vi "Actor Core.vi"(8 "error in":errorcluster, 11 "Panel in":refnum<class "Sample Panel.lvclass">) -> (0 "error out":errorcluster, 3 "Actor out":refnum<class "Actor.lvclass">)   [LabVIEW 2020, in "2. Basic Panel Actors.lvlib" / "Sample Panel.lvclass"]
doc: "Shows the Label and a log of all events for the panel.\n----\nCopyright: MGI 2016\nAuthor: Derek Trepanier"
uses:
  Sample Panel.lvclass
  C:/Program Files/National Instruments/LabVIEW 2020/vi.lib/MGI/Monitored Actor/Monitored Actor/Monitored Actor/Monitored Actor.lvclass
  C:/Program Files/National Instruments/LabVIEW 2020/vi.lib/MGI/Panel Manager/Panel Actor/Panel Actor/Panel Actor.lvclass
  <vilib>/ActorFramework/Actor/Actor.lvclass
  <vilib>/ActorFramework/Message Enqueuer/Message Enqueuer.lvclass/Message Enqueuer.ctl
  <vilib>/ActorFramework/Message Enqueuer/Enqueue.vi
  <vilib>/ActorFramework/Stop Msg/Stop Msg.lvclass
  C:/Program Files/National Instruments/LabVIEW 2020/vi.lib/ActorFramework/Message/Message.lvclass
  <vilib>/ActorFramework/Message Priority Queue/Priority Enqueue.vi
  <vilib>/MGI/Panel Manager/Panel Actor/Panel Actor/Panel Actor.lvclass
  <vilib>/MGI/Monitored Actor/Monitored Actor/Monitored Actor/Monitored Actor.lvclass
panel:
  out "Label":string
  out "Top Level Panel":string
  in  "Show":bool
  in  "My Event Log":i32(listbox)
  in  "Show Dialog":bool
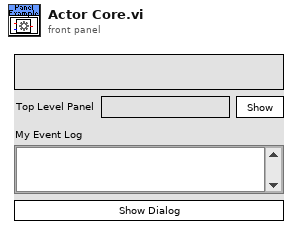
[diagram p1: front panel]
types:
  T1 = typedef "Panel.lvlib/Panel Helper.lvclass/Events.ctl" = enum16{"Initialized", "Shown", "Hidden", "Closed"}
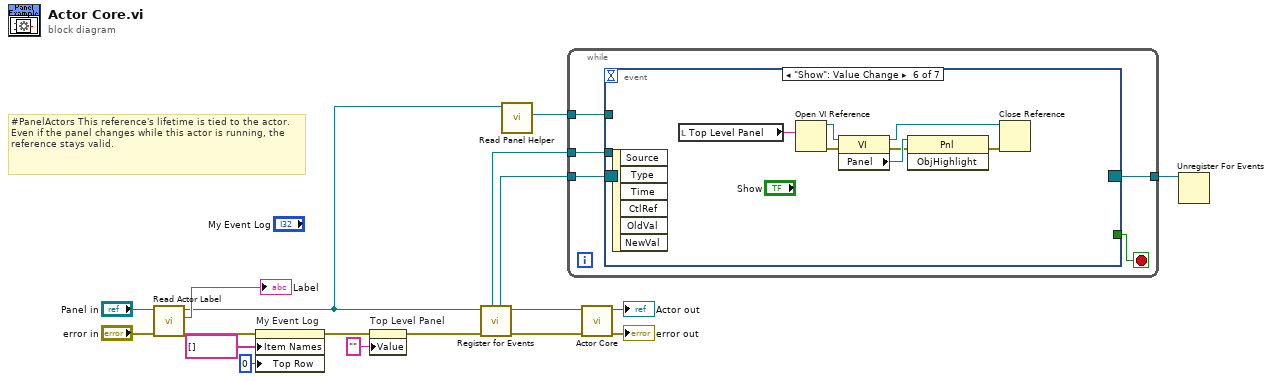
[diagram p0: block diagram]
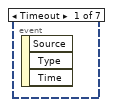
[diagram p2: hidden frame]
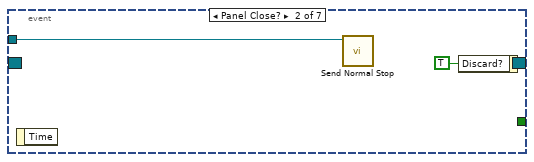
[diagram p3: hidden frame]
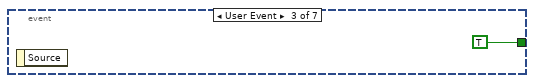
[diagram p4: hidden frame]
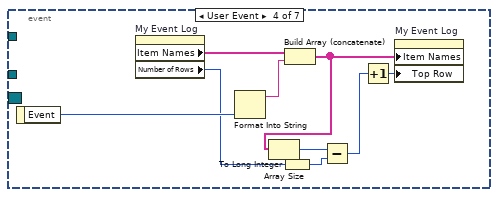
[diagram p5: hidden frame]
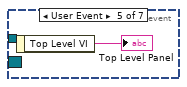
[diagram p6: hidden frame]
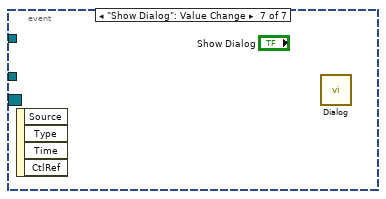
[diagram p7: hidden frame]
diagram:
  # "#PanelActors This reference's lifetime is tied to the actor. Even if the panel changes while this actor is running, the reference stays valid."
  n1 = call <vilib>:"Read Actor Label.vi"("error in (no error)"="error in", "Monitored Actor in"="Panel in") -> ("error out"=w11:errorcluster, "Actor Label"=→"Label":string, "Monitored Actor out"=w8:refnum<class "Sample Panel.lvclass">)  [unwired: 7 in]
  n2 = property on="My Event Log" class="LstBox (strict)"(error in=w11, "Item Names"=string[] [], "Top Row"=0) -> (error out=w3:errorcluster)  [unwired: 1 in, 1 out]
  n3 = property on="Top Level Panel" class="Str"(error in=w3, "Value"="" ("Top Level Panel")) -> (error out=w2:errorcluster)  [unwired: 1 in, 1 out]
  n4 = call <vilib>:"Register for Events.vi"("Error In"=w2, "Panel Actor in"=w8) -> ("Error Out"=w9:errorcluster, "Panel Actor out"=w13:refnum<class "Sample Panel.lvclass">, "Pnl Actor"=w10:refnum<event-registration>, "Self Enqueuer"=w12:refnum<class "Message Enqueuer.lvclass">)  [unwired: 6 in]
  n5 = call <vilib>:"Read Panel Helper.vi"("Panel Actor in"=w8) -> ("Panel Helper"=w7:refnum<class "Panel Helper.lvclass">)  [unwired: 9 in, 1 out]
  n6 = while {
    tunnel: w12 -> [w23]
    tunnel: w10 -> [w22]
    tunnel: w7 -> [w20]
    tunnel: [w19] -> w6
    stop <- w21 stop-if-true
    n7 = event shown="[5] \"Show\": Value Change" {
      selector: w22 -> [_ _ _ _ _ _ _]
      dyn-events: [_ _ _ _ _ _ _] -> w19
      timeout: _ -> [_ _ _ _ _ _ _]
      tunnel: w23 -> [_ w24 _ _ _ _ _]
      tunnel: [_ _ TRUE _ _ _ _] -> w21
      tunnel: w20 -> [_ _ _ _ _ _ _]
      event Timeout {
        n8 = event-data() -> ()  [unwired: 1 in, 3 out]
      }
      event Panel Close? {
        n9 = event-data() -> ()  [unwired: 1 in, 1 out]
        n10 = call <vilib>:"Send Normal Stop.vi"("Message Enqueuer"=w24) -> ()  [unwired: 10 in, 1 out]
        n11 = event-data("Discard?"=TRUE) -> ()  [unwired: 1 in, 1 out]
      }
      event User Event {
        n12 = event-data() -> ()  [unwired: 1 in, 1 out]
      }
      event User Event {
        n13 = event-data() -> ("Event"=w34:T1)  [unwired: 1 in]
        n14 = property on="My Event Log" class="LstBox (strict)"() -> ("Item Names"=w33:string[], "Number of Rows"=w31:u32)  [unwired: 2 in, 2 out]
        n15 = Format Into String(w34) -> (resulting string=w35:string)  [unwired: 3 in, 1 out]
        n16 = To Long Integer(number=w31) -> (32bit integer=w27:i32)
        n17 = Build Array (concatenate)(w33, w35) -> (w29:string[])
        n18 = Array Size(array=w29) -> (size(s)=w32:i32)
        n19 = Subtract(x=w32, y=w27) -> (x-y=w30:i32)
        n20 = Increment(x=w30) -> (x+1=w28:i32)
        n21 = property on="My Event Log" class="LstBox (strict)"("Item Names"=w29, "Top Row"=w28) -> ()  [unwired: 2 in, 2 out]
      }
      event User Event {
        n22 = event-data() -> ("Top Level VI"=→"Top Level Panel":string)  [unwired: 1 in]
      }
      event "Show": Value Change {
        n23 = event-data() -> ()  [unwired: 1 in, 6 out]
        n24 = local read "Top Level Panel"() -> (w43:string)
        n25 = Open VI Reference(vi path=w43) -> (vi reference=w42:refnum<vi>, error out=w39:errorcluster)  [unwired: 5 in]
        n26 = property class="VI"(reference=w42, error in=w39) -> (reference out=w41:refnum<vi>, error out=w38:errorcluster, "Panel"=w40:refnum<vi>)
        n27 = invoke class="Pnl" method="ObjHighlight"(reference=w40, error in=w38) -> (error out=w37:errorcluster)  [unwired: 1 in, 2 out]
        n28 = Close Reference(reference=w41, error in (no error)=w37) -> ()  [unwired: 1 out]
      }
      event "Show Dialog": Value Change {
        n29 = event-data() -> ()  [unwired: 1 in, 4 out]
        n30 = call "Dialog.vi"() -> ()  [unwired: 12 in]
      }
    }
  }
  n31 = call-parent "Actor Core.vi"("error in"=w9, "Panel Actor in"=w13) -> ("error out"=→"error out":errorcluster, "Actor out"=→"Actor out":refnum<class "Actor.lvclass">)  [unwired: 8 in]
  n32 = Unregister For Events(event registration refnum=w6) -> ()  [unwired: 1 in, 1 out]
